vi "Refresh Routes.vi"(8 "error in (no error)":errorcluster, 11 "MuxPanel in":refnum<class "MuxPanel.lvclass">) -> (0 "error out":errorcluster, 3 "MuxPanel out":refnum<class "MuxPanel.lvclass">)   [LabVIEW 2022 SP3, in "TouchControl.lvlib" / "MuxPanel.lvclass"]
uses:
  MuxPanel.lvclass
  MuxPanel.lvclass/MuxPanel.ctl
  TouchControl.lvlib
  <vilib>/httpClient/LabVIEWHTTPClient.lvlib
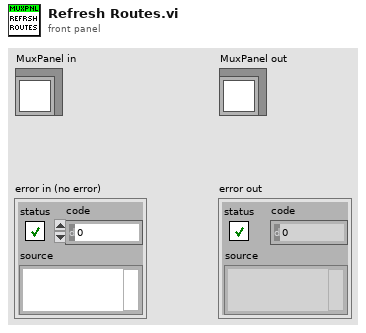
[diagram p1: front panel]
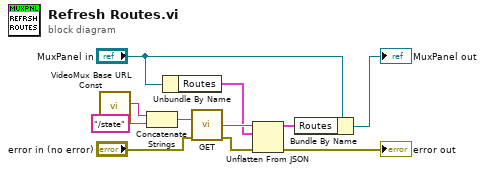
[diagram p0: block diagram]
diagram:
  n1 = call "VideoMux Base URL Const.vi"() -> ("VideoMux Base URL"=w11:string)  [unwired: 11 in]
  n2 = Concatenate Strings(w11, "/state" ("string")) -> (w9:string)
  n3 = Unbundle By Name("MuxPanel in") -> ("Routes"=w7:cluster{"Mux Route":i32[]}[])
  n4 = call <vilib>:"GET.vi"("url"=w9, "error in (no error)"="error in (no error)") -> ("body"=w8:string, "error out"=w3:errorcluster)  [unwired: 10 in, 2 out]
  n5 = Unflatten From JSON(JSON string=w8, type and defaults=w7, error in (no error)=w3) -> (value=w6:cluster{"Mux Route":i32[]}[], error out=→"error out":errorcluster)  [unwired: 4 in]
  n6 = Bundle By Name(cluster="MuxPanel in", "Routes"=w6) -> (→"MuxPanel out":refnum<class "MuxPanel.lvclass">)
